vi "convert b&w to color map.vi"(5 "Image":T1) -> (2 "colored":T1(plugin-control))   [LabVIEW 2012]
uses:
  <vilib>/vision/Image Controls.llb/IMAQ Image.ctl
  <vilib>/vision/NI_Vision_Development_Module.lvlib
panel:
  out "Original":T1(plugin-control)
  out "Converted":T1(plugin-control)
  in  "Palette Number (gray)":T2(ring)
  # "labview"
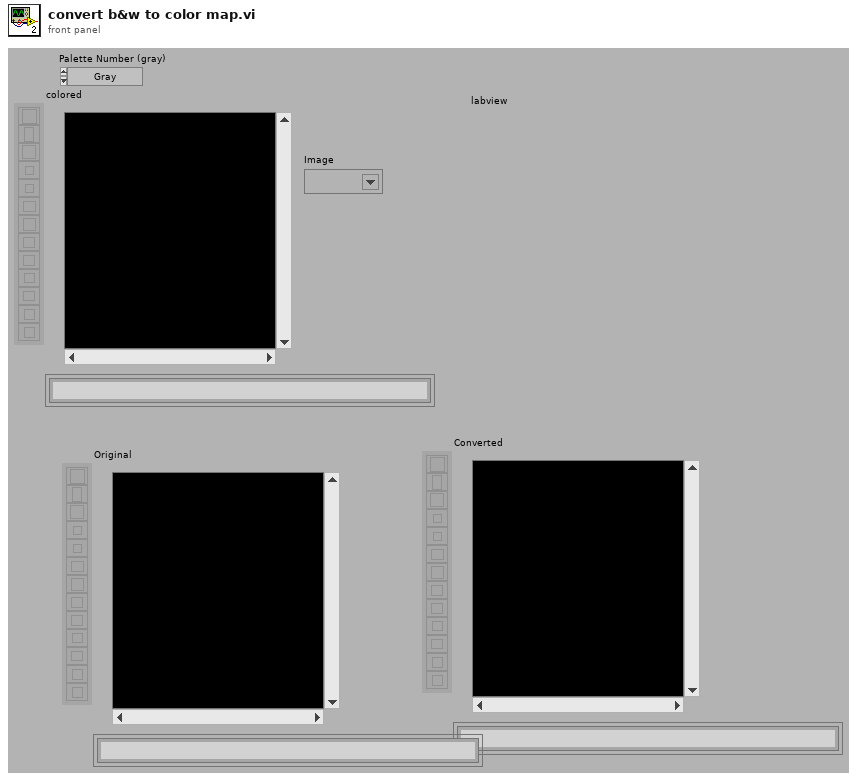
[diagram p1: front panel]
types:
  T1 = typedef "IMAQ Image.ctl" = refnum<image>
  T2 = enum32{"Gray", "Binary", "Gradient", "Rainbow", "Temperature"}
  T3 = typedef "Image Type" = u32
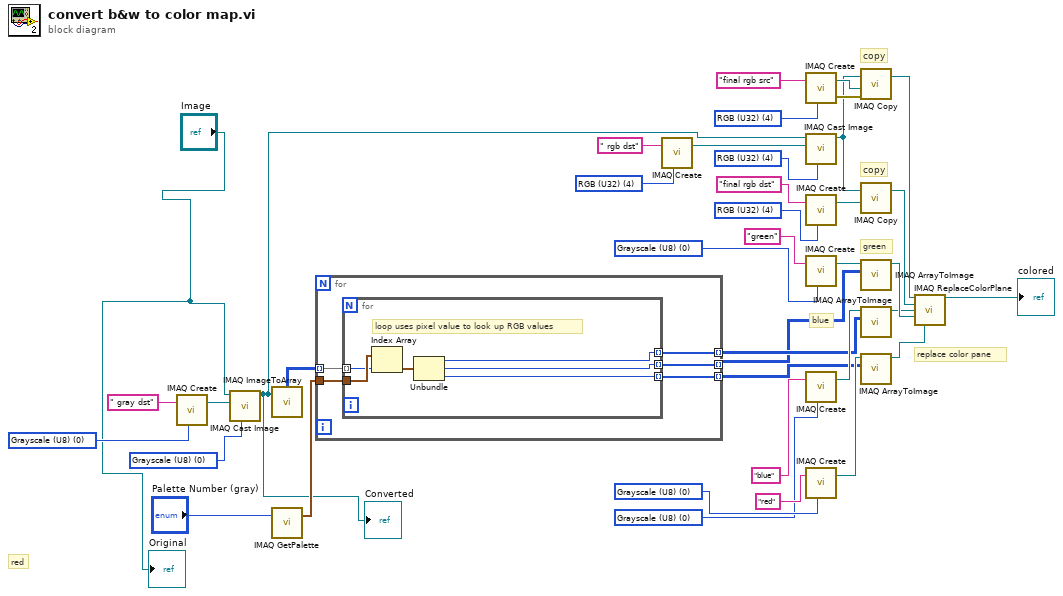
[diagram p0: block diagram]
diagram:
  w5 = T3 0 items=["Grayscale (U8)", "Grayscale (I16)", "Grayscale (SGL)", "Complex (CSG)", "RGB (U32)", "HSL (U32)", "RGB (U64)", "Grayscale (U16)"] ("Image Type")
  w7 = T3 4 items=["Grayscale (U8)", "Grayscale (I16)", "Grayscale (SGL)", "Complex (CSG)", "RGB (U32)", "HSL (U32)", "RGB (U64)", "Grayscale (U16)"] ("Image Type")
  w10 = T3 4 items=["Grayscale (U8)", "Grayscale (I16)", "Grayscale (SGL)", "Complex (CSG)", "RGB (U32)", "HSL (U32)", "RGB (U64)", "Grayscale (U16)"] ("Image Type")
  w11 = T3 0 items=["Grayscale (U8)", "Grayscale (I16)", "Grayscale (SGL)", "Complex (CSG)", "RGB (U32)", "HSL (U32)", "RGB (U64)", "Grayscale (U16)"] ("Image Type")
  w29 = T3 0 items=["Grayscale (U8)", "Grayscale (I16)", "Grayscale (SGL)", "Complex (CSG)", "RGB (U32)", "HSL (U32)", "RGB (U64)", "Grayscale (U16)"] ("Image Type")
  w32 = T3 0 items=["Grayscale (U8)", "Grayscale (I16)", "Grayscale (SGL)", "Complex (CSG)", "RGB (U32)", "HSL (U32)", "RGB (U64)", "Grayscale (U16)"] ("Image Type")
  w33 = T3 0 items=["Grayscale (U8)", "Grayscale (I16)", "Grayscale (SGL)", "Complex (CSG)", "RGB (U32)", "HSL (U32)", "RGB (U64)", "Grayscale (U16)"] ("Image Type")
  w36 = T3 4 items=["Grayscale (U8)", "Grayscale (I16)", "Grayscale (SGL)", "Complex (CSG)", "RGB (U32)", "HSL (U32)", "RGB (U64)", "Grayscale (U16)"] ("Image Type")
  w38 = T3 4 items=["Grayscale (U8)", "Grayscale (I16)", "Grayscale (SGL)", "Complex (CSG)", "RGB (U32)", "HSL (U32)", "RGB (U64)", "Grayscale (U16)"] ("Image Type")
  # "replace color pane"
  # "copy"
  # "copy"
  # "red"
  # "green"
  # "blue"
  n1 = call "IMAQ Create"("Image Name"=" gray dst", "Image Type"=w5) -> ("New Image"=w3:T1)  [unwired: 2 in, 2 out]
  n2 = call "IMAQ Cast Image"("Image Type"=w11, "Image Dst"=w3, "Image Src"="Image") -> ("Image Dst Out"=w2:T1)  [unwired: 7 in, 1 out]
  "Converted" <- w2
  n3 = call "IMAQ ImageToArray"("Image"=w2) -> ("Image Pixels (U8)"=w16:u8[][])  [unwired: 2 in, 5 out]
  n4 = call "IMAQ GetPalette"("Palette Number (gray)"="Palette Number (gray)") -> ("Color Palette"=w37:cluster{"Red":u8, "Green":u8, "Blue":u8}[])  [unwired: 1 in, 4 out]
  n5 = for {
    tunnel: w37 -> [w44]
    tunnel: w16 -> [w43] mode=indexing
    tunnel: [w42] -> w25 mode=indexing
    tunnel: [w41] -> w24 mode=indexing
    tunnel: [w40] -> w23 mode=indexing
    n6 = for {
      tunnel: w44 -> [w50]
      tunnel: w43 -> [w48] mode=indexing
      tunnel: [w47] -> w42 mode=indexing
      tunnel: [w46] -> w41 mode=indexing
      tunnel: [w45] -> w40 mode=indexing
      # "loop uses pixel value to look up RGB values"
      n7 = Index Array(array=w50, index=w48) -> (element=w49:cluster{"Red":u8, "Green":u8, "Blue":u8})
      n8 = Unbundle(w49) -> ("Red"=w47:u8, "Green"=w46:u8, "Blue"=w45:u8)
    }
  }
  n9 = call "IMAQ Create"("Image Name"=" rgb dst", "Image Type"=w7) -> ("New Image"=w6:T1)  [unwired: 2 in, 2 out]
  n10 = call "IMAQ Create"("Image Name"="final rgb src", "Image Type"=w38) -> ("New Image"=w20:T1, "error out"=w21:errorcluster)  [unwired: 2 in, 1 out]
  n11 = call "IMAQ Cast Image"("Image Type"=w10, "Image Dst"=w6, "Image Src"=w2) -> ("Image Dst Out"=w9:T1)  [unwired: 7 in, 1 out]
  n12 = call "IMAQ Create"("Image Name"="final rgb dst", "Image Type"=w36) -> ("New Image"=w19:T1)  [unwired: 2 in, 2 out]
  n13 = call "IMAQ Create"("Image Name"="green", "Image Type"=w32) -> ("New Image"=w27:T1)  [unwired: 2 in, 2 out]
  n14 = call "IMAQ Create"("Image Name"="blue", "Image Type"=w29) -> ("New Image"=w26:T1)  [unwired: 2 in, 2 out]
  n15 = call "IMAQ Create"("Image Name"="red", "Image Type"=w33) -> ("New Image"=w28:T1)  [unwired: 2 in, 2 out]
  n16 = call "IMAQ Copy"("error in (no error)"=w21, "Image Dst"=w20, "Image Src"=w9) -> ("Image Dst Out"=w17:T1)  [unwired: 4 out]
  n17 = call "IMAQ Copy"("Image Dst"=w19, "Image Src"=w9) -> ("Image Dst Out"=w18:T1)  [unwired: 1 in, 4 out]
  n18 = call "IMAQ ArrayToImage"("Image Pixels (U8)"=w24, "Image"=w27) -> ("Image Out"=w22:T1)  [unwired: 4 in, 5 out]
  n19 = call "IMAQ ArrayToImage"("Image Pixels (U8)"=w25, "Image"=w26) -> ("Image Out"=w14:T1)  [unwired: 4 in, 5 out]
  n20 = call "IMAQ ArrayToImage"("Image Pixels (U8)"=w23, "Image"=w28) -> ("Image Out"=w15:T1)  [unwired: 4 in, 5 out]
  n21 = call "IMAQ ReplaceColorPlane"("Image Src"=w17, "Image Dst"=w18, "Red or Hue Plane"=w14, "Green or Sat Plane"=w22, "Blue or Luma or Val or Inten Plane"=w15) -> ("Image Dst Out"=→"colored":T1)  [unwired: 2 in, 8 out]
  "Original" <- "Image"
